vi "Definitions Tester.vi"() -> ()   [LabVIEW 2023]
uses:
  Defintion FGV Actions.ctl
  JSON Schema Generator.lvlib
  <vilib>/JDP Science/JSONtext/JSONtext.lvlib
panel:
  in  "Action":T1
  in  "Defintion Schema":string
  in  "Definition Name":string
  out "<JSON>":string caption="<JSON>First JSON Value"
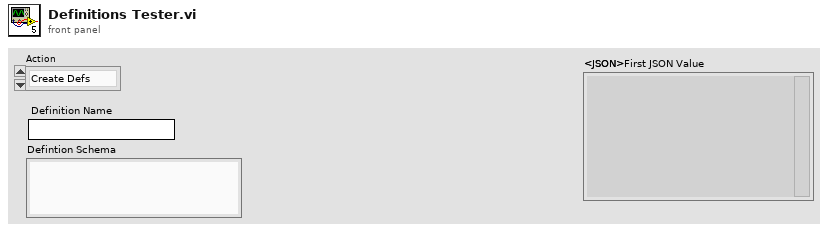
[diagram p1: front panel]
types:
  T1 = typedef "JSON Schema Generator.lvlib/Defintion FGV Actions.ctl" = enum16{"Create Defs", "Update Defs", "Get all Defs", "Get Def"}
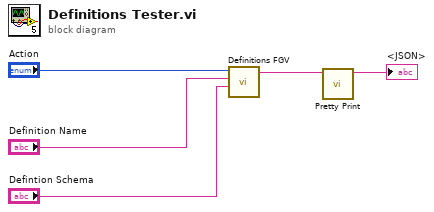
[diagram p0: block diagram]
diagram:
  n1 = call "Definitions FGV.vi"("Defintion Schema In"="Defintion Schema", "Definition Name"="Definition Name", "Action"="Action") -> ("Definitions out"=w5:string)  [unwired: 7 in, 1 out]
  n2 = call <vilib>:"Pretty Print.vi"("JSON"=w5) -> ("<JSON>"=→"<JSON>":string)  [unwired: 8 in, 2 out]
